vi "Shiftregister.vi"() -> ()   [LabVIEW 2019]
panel:
  out "Factorial":i32
  in  "Number":i32
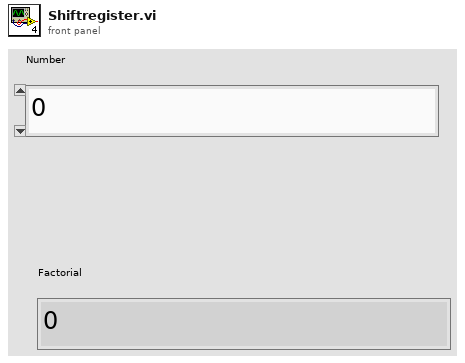
[diagram p1: front panel]
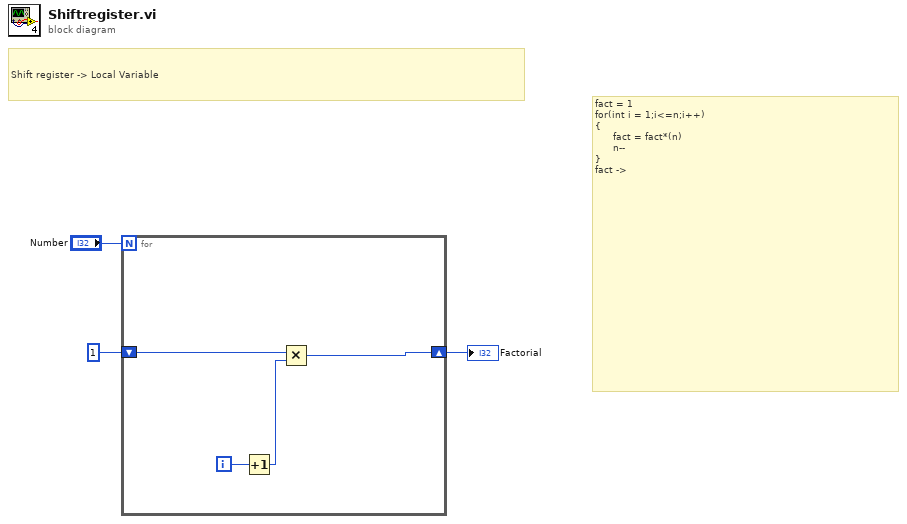
[diagram p0: block diagram]
diagram:
  # "fact = 1\nfor(int i = 1;i<=n;i++)\n{\n      fact = fact*(n)\n      n--\n}\nfact ->"
  # "Shift register -> Local Variable"
  n1 = for {
    N: "Number" -> [_]
    shift-right: [w4] -> w1
    shift-left: 1 ("x") -> [w5]
    i -> [w7]
    n2 = Increment(x=w7) -> (x+1=w6:i32)
    n3 = Multiply(x=w5, y=w6) -> (x*y=w4:i32)
  }
  "Factorial" <- w1
